vi "ClassPanel.vi"(8 "error in (no error)":errorcluster caption="entrée d'erreur (pas d'erreur)", 11 "ThorKDC101.lvclass":refnum<class "ThorKDC101.lvclass">) -> (0 "error out":errorcluster caption="sortie d'erreur", 3 "ThorKDC101.lvclass Out":refnum<class "ThorKDC101.lvclass">)   [LabVIEW 2019, in "ThorKDC101.lvclass"]
uses:
  ThorKDC101.lvclass
  C:/Programmes Labview/LabScanV1A/DevicesClass/BaseDevice/BaseDevice.lvclass
  BaseDevice/ClassQueueMess.ctl
  ThorKDC101.lvclass/ThorKDC101.ctl
  BaseDevice/Accessor/GetClassEvent.vi
panel:
  in  "Home":bool caption="MiseAJour"
  out "ActPos(Deg)":dbl=60.0 caption="ActPos(deg)" min=0.1 step=0.1 format="%#.1f"
  in  "Con/Disc.":bool
  out "InstrName":string
  out "Homed":bool
  out "Moving":bool
  in  "MainProgQ":refnum<queue>
  in  "MainProgQEvent":refnum<user-event>
  in  "Acq":bool
  in  "Stop":bool
  in  "StopMove":bool caption="MiseAJour"
  in  "Position(Deg)":dbl=60.0 caption="Position(deg)" format="%#.1f"
  out "Init Program":bool
  # "this MUST labeled with class name"
  # "this MUST be present and labeled \"Stop\" and \"Acq\""
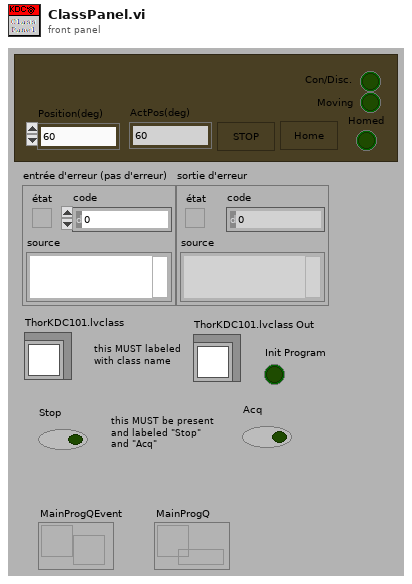
[diagram p1: front panel]
types:
  T1 = typedef "ClassQueueMess.ctl" = u16
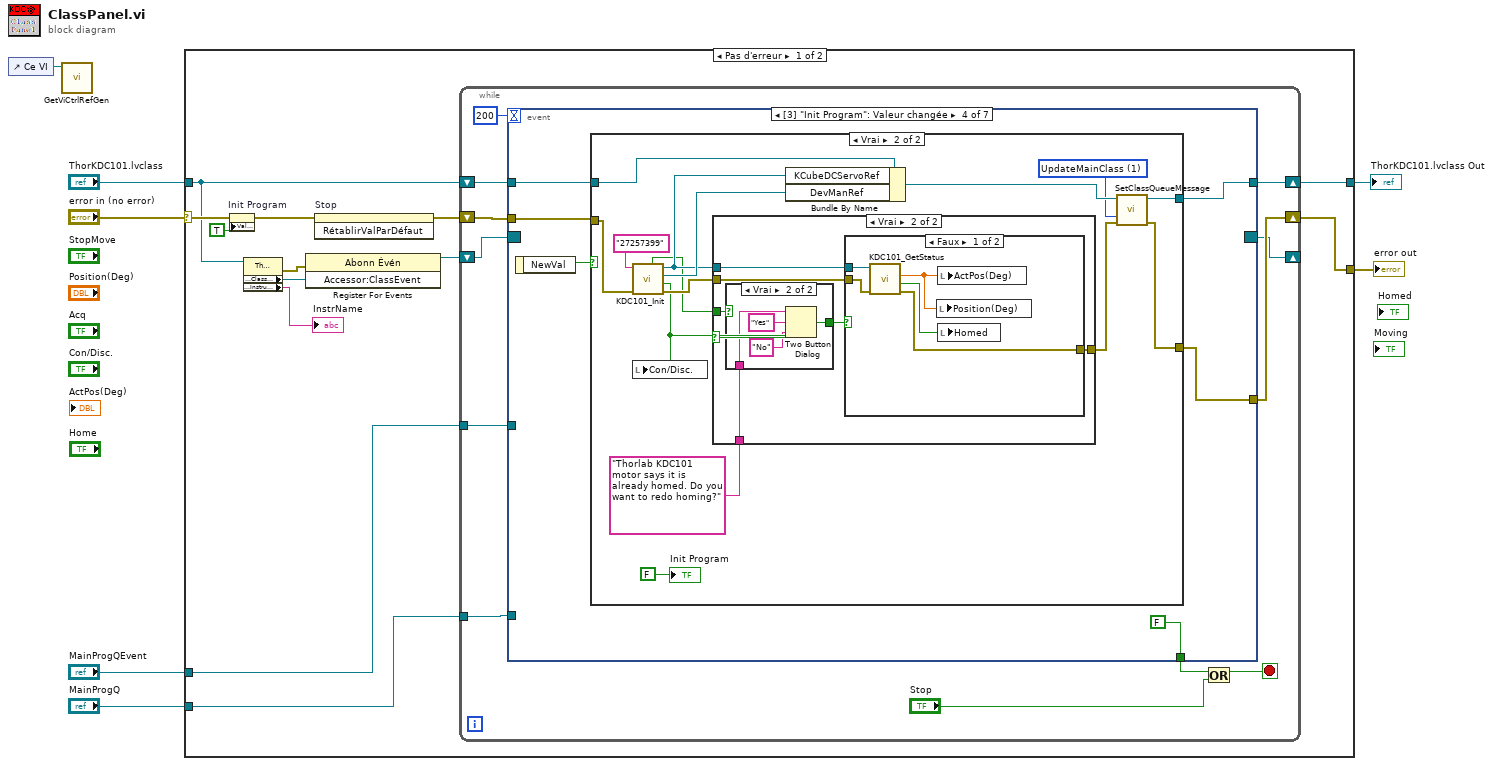
[diagram p0: block diagram]
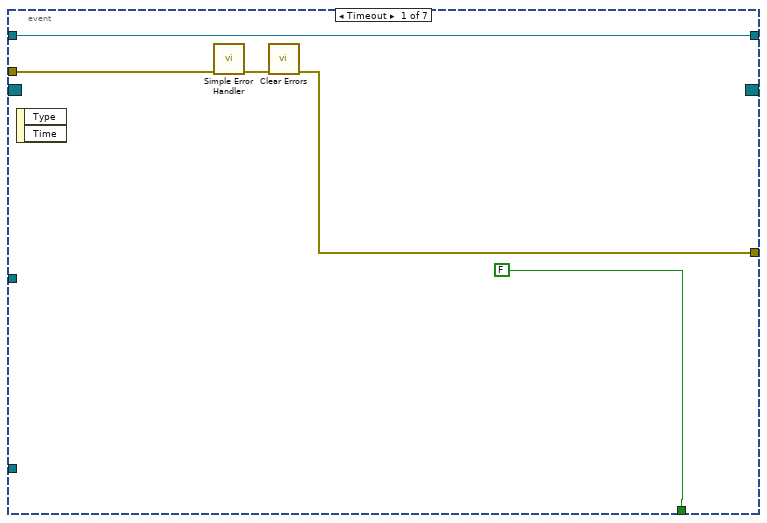
[diagram p2: hidden frame]
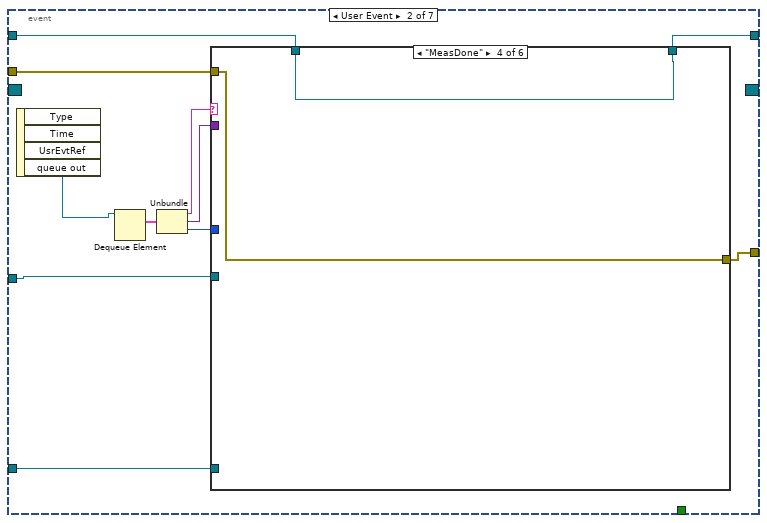
[diagram p3: hidden frame]
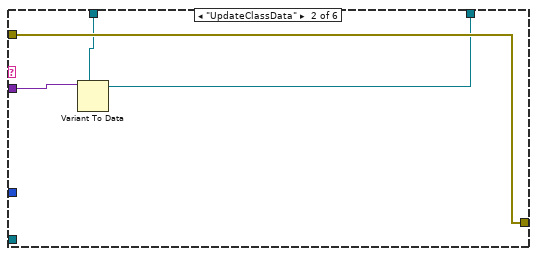
[diagram p5: hidden frame]
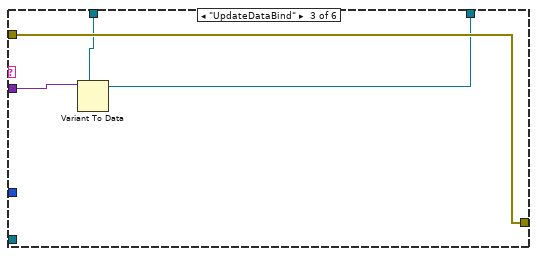
[diagram p6: hidden frame]
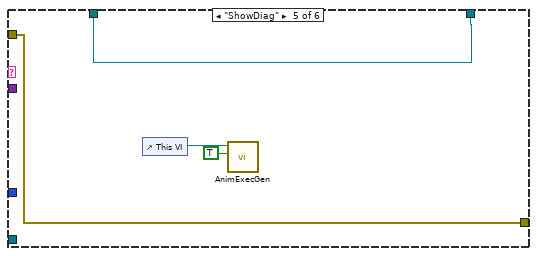
[diagram p7: hidden frame]
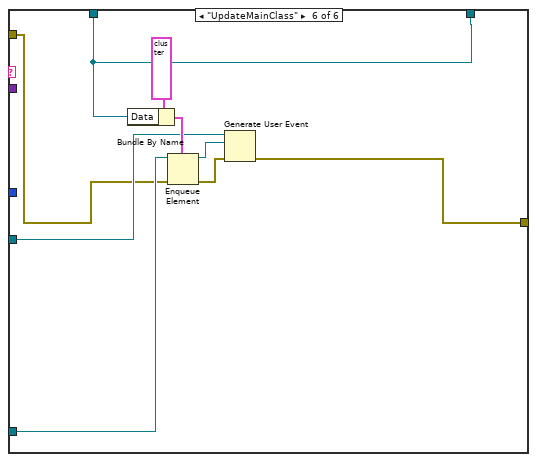
[diagram p8: hidden frame]
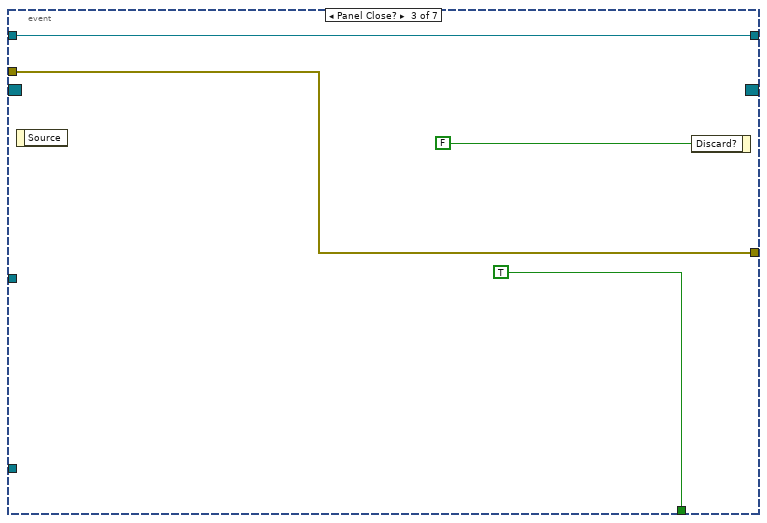
[diagram p9: hidden frame]
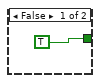
[diagram p12: hidden frame]
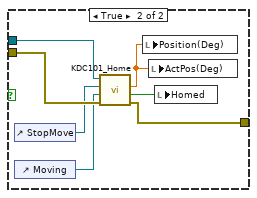
[diagram p13: hidden frame]
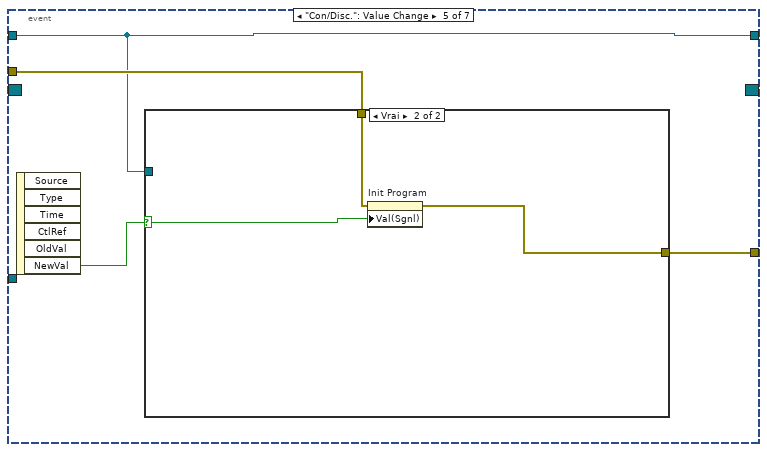
[diagram p14: hidden frame]
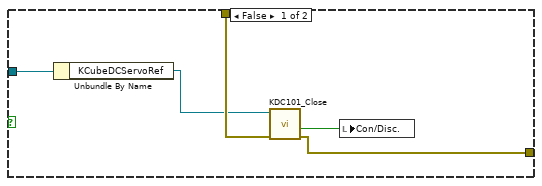
[diagram p15: hidden frame]
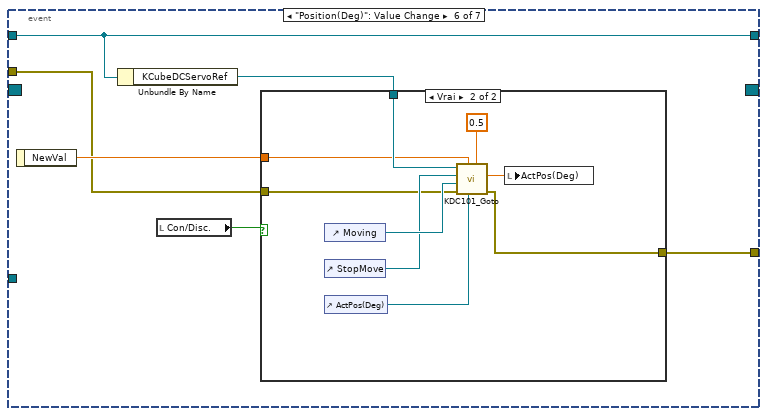
[diagram p16: hidden frame]
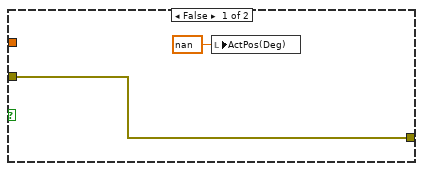
[diagram p17: hidden frame]
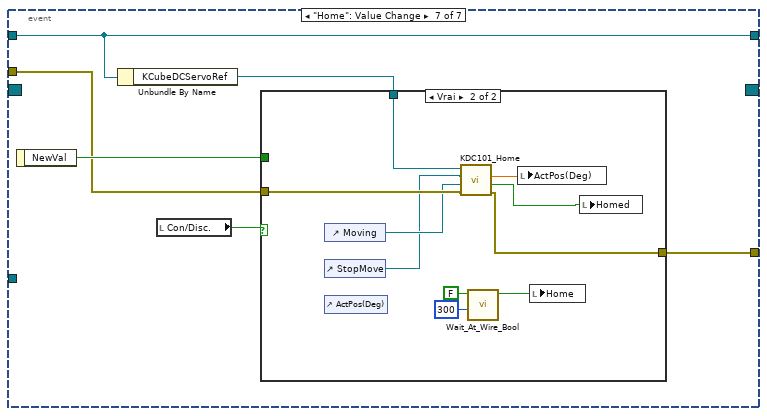
[diagram p18: hidden frame]
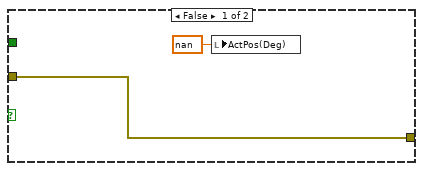
[diagram p19: hidden frame]
diagram:
  n1 = control-ref of="Ce VI"() -> (w1:refnum<vi>)
  n2 = call <userlib>:"GetViCtrlRefGen.vi"("VIRef"=w1) -> ()  [unwired: 8 in, 3 out]
  n3 = case shown="Pas d'erreur" "error in (no error)" {
    selector: "error in (no error)" -> [w17 w173]
    tunnel: [w20 w173] -> w6
    tunnel: "ThorKDC101.lvclass" -> [w12 w172]
    tunnel: [w18 w172] -> w4
    tunnel: "MainProgQEvent" -> [w10 _]
    tunnel: "MainProgQ" -> [w9 _]
    frame No Error {
      n4 = property on="Init Program" class="Bool (strict)"(error in=w17, "Val(Sgnl)"=TRUE ("Valeur (Signalisation)")) -> (error out=w16:errorcluster)  [unwired: 1 in, 1 out]
      n5 = property class="ThorKDC101.lvclass"(reference=w12) -> (error out=w14:errorcluster, "Accessor:ClassEvent"=w13:refnum<user-event>, "Accessor:InstrumentName"=→"InstrName":string)  [unwired: 1 in, 1 out]
      n6 = register-events(error in=w14, w13) -> (reference out=w11:refnum<event-registration>)  [unwired: 1 in, 1 out]
      n7 = invoke on="Stop" class="Bool (strict)" method="RétablirValParDéfaut"(error in=w16) -> (error out=w15:errorcluster)  [unwired: 2 in, 2 out]
      n8 = while {
        shift-right: [w30] -> w20
        shift-left: w15 -> [w31]
        shift-right: [w27] -> w18
        shift-left: w12 -> [w29]
        shift-right: [w23] -> _
        shift-left: w11 -> [w24]
        tunnel: w10 -> [w22]
        tunnel: w9 -> [w21]
        stop <- w26 stop-if-true
        n9 = event shown="[3] \"Init Program\": Valeur changée" {
          selector: w24 -> [_ _ _ _ _ _ _]
          dyn-events: [_ _ _ _ _ _ _] -> w23
          timeout: 200 -> [_ _ _ _ _ _ _]
          tunnel: w31 -> [w35 w47 w75 w82 w127 w139 w156]
          tunnel: [w33 w41 w75 w79 w126 w138 w155] -> w30
          tunnel: w29 -> [w36 w48 w74 w80 w125 w142 w159]
          tunnel: [FALSE _ TRUE FALSE _ _ _] -> w28
          tunnel: [w36 w40 w74 w78 w125 w142 w159] -> w27
          tunnel: w22 -> [_ w39 _ _ _ _ _]
          tunnel: w21 -> [_ w38 _ _ _ _ _]
          event Timeout {
            n10 = event-data() -> ()  [unwired: 1 in, 2 out]
            n11 = call <vilib>:"Simple Error Handler.vi"("error in (no error)"=w35) -> ("error out"=w34:errorcluster)  [unwired: 4 in, 4 out]
            n12 = call <vilib>:"Clear Errors.vi"("error in (no error)"=w34) -> ("error out"=w33:errorcluster)  [unwired: 5 in, 1 out]
          }
          event User Event {
            n13 = event-data() -> ("queue out"=w45:refnum<queue>)  [unwired: 1 in, 3 out]
            n14 = Dequeue Element(queue=w45) -> (element=w46:cluster{"Message":string, "Data":variant, i32})  [unwired: 2 in, 3 out]
            n15 = Unbundle(w46) -> ("Message"=w44:string, "Data"=w43:variant, w42:i32)
            n16 = case shown="\"MeasDone\"" w44 {
              tunnel: w47 -> [w50 w54 w58 w59 w63 w66]
              tunnel: w43 -> [_ w53 w57 _ _ _]
              tunnel: w48 -> [w49 w52 w56 w60 w64 w69]
              tunnel: [w49 w51 w55 w60 w64 w69] -> w40
              tunnel: [w50 w54 w58 w59 w63 w65] -> w41
              tunnel: w42 -> [_ _ _ _ _ _]
              tunnel: w39 -> [_ _ _ _ _ w68]
              tunnel: w38 -> [_ _ _ _ _ w67]
              frame Default {
              }
              frame "UpdateClassData" {
                n17 = Variant To Data(type=w52, Variant=w53) -> (data=w51:refnum<class "ThorKDC101.lvclass">)  [unwired: 1 in, 1 out]
              }
              frame "UpdateDataBind" {
                n18 = Variant To Data(type=w56, Variant=w57) -> (data=w55:refnum<class "ThorKDC101.lvclass">)  [unwired: 1 in, 1 out]
              }
              frame "MeasDone" {
              }
              frame "ShowDiag" {
                n19 = control-ref of="This VI"() -> (w62:refnum<vi>)
                n20 = call <userlib>:"AnimExecGen.vi"("Animer l'exécution ?"=TRUE, "ViRef"=w62) -> ()  [unwired: 9 in, 1 out]
              }
              frame "UpdateMainClass" {
                n21 = Bundle By Name(cluster=cluster{"Message":string, "Data":variant, i32} {"Message"="", "Data"=variant, 0} ("élément"), "Data"=w69) -> (w70:cluster{"Message":string, "Data":variant, i32})
                n22 = Enqueue Element(queue=w67, element=w70, error in (no error)=w66) -> (queue out=w73:refnum<queue>, error out=w72:errorcluster)  [unwired: 1 in, 1 out]
                n23 = Generate User Event(user event=w68, event data cluster=w73, error in=w72) -> (error out=w65:errorcluster)  [unwired: 1 in, 1 out]
              }
            }
          }
          event Panel Close? {
            n24 = event-data() -> ()  [unwired: 1 in, 1 out]
            n25 = event-data("Discard?"=FALSE ("Rejeter ?")) -> ()  [unwired: 1 in, 1 out]
          }
          event "Init Program": Value Change {
            n26 = event-data() -> ("NewVal"=w83:bool)  [unwired: 1 in]
            n27 = case shown="Vrai" w83 {
              tunnel: w82 -> [w85 w95]
              tunnel: [w85 w94] -> w79
              tunnel: w80 -> [w84 w89]
              tunnel: [w84 w93] -> w78
              frame False {
              }
              frame True {
                w96 = T1 1 items=["UpdateClassData", "UpdateMainClass", "UpdateDataBind", "ReInitDevice", "Custom", "ClosePan"] ("Menu déroulant")
                n28 = call <userlib>:"KDC101_Init.vi"("error in (no error)"=w95, "serialNo"="27257399") -> ("error out"=w92:errorcluster, "Connected"=w88:bool, "DevManRef"=w98:refnum<k24>, "KCubeDCServoRef"=w91:refnum<k24>, "IsHomed"=w87:bool)  [unwired: 4 in, 1 out]
                n29 = local write "Con/Disc."(w88) -> ()
                n30 = case shown="Vrai" w88 {
                  tunnel: w92 -> [w101 w107]
                  tunnel: w91 -> [_ w106]
                  tunnel: [w101 w105] -> w90
                  tunnel: w87 -> [_ w102]
                  tunnel: "Thorlab KDC101 motor says it is already homed. Do you want to redo homing?" -> [_ w103]
                  frame False {
                  }
                  frame True {
                    n31 = case shown="Vrai" w102 {
                      tunnel: [TRUE w112] -> w104
                      tunnel: w103 -> [_ w111]
                      frame False {
                      }
                      frame True {
                        n32 = Two Button Dialog(message=w111, 1:"No" ("Nom du bouton F (\"Annuler\")"), 2:"Yes" ("Nom du bouton V (\"OK\")")) -> (T button?=w112:bool)
                      }
                    }
                    n33 = case shown="Faux" w104 {
                      tunnel: w107 -> [w116 w124]
                      tunnel: w106 -> [w117 w121]
                      tunnel: [w115 w119] -> w105
                      frame False {
                        n34 = call <userlib>:"KDC101_GetStatus.vi"("error in (no error)"=w116, "KCubeDCServoRef"=w117) -> ("error out"=w115:errorcluster, "Homed"=w114:bool, "ActPos(Deg)"=w113:dbl)  [unwired: 5 in, 2 out]
                        n35 = local write "Position(Deg)"(w113) -> ()
                        n36 = local write "ActPos(Deg)"(w113) -> ()
                        n37 = local write "Homed"(w114) -> ()
                      }
                      frame True {
                        n38 = control-ref of="StopMove"() -> (w122:refnum<vi>)
                        n39 = control-ref of="Moving"() -> (w123:refnum<vi>)
                        n40 = call <userlib>:"KDC101_Home.vi"("error in (no error)"=w124, "MovingRef"=w123, "StopRef"=w122, "KCubeDCServoRef"=w121) -> ("error out"=w119:errorcluster, "Homed"=w120:bool, "ActPos(Deg)"=w118:dbl)  [unwired: 4 in, 1 out]
                        n41 = local write "Position(Deg)"(w118) -> ()
                        n42 = local write "ActPos(Deg)"(w118) -> ()
                        n43 = local write "Homed"(w120) -> ()
                      }
                    }
                  }
                }
                n44 = Bundle By Name(cluster=w89, "KCubeDCServoRef"=w91, "DevManRef"=w98) -> (w97:refnum<class "ThorKDC101.lvclass">)
                n45 = call-dynamic "SetClassQueueMessage.vi"("ErrorIn(No Error)"=w90, "Menu déroulant"=w96, "DefaultDev.lvclass"=w97) -> ("sortie d'erreur"=w94:errorcluster, "DefaultDev.lvclass Out"=w93:refnum<class "ThorKDC101.lvclass">)  [unwired: 7 in]
                "Init Program" <- FALSE
              }
            }
          }
          event "Con/Disc.": Value Change {
            n46 = event-data() -> ("NewVal"=w128:bool)  [unwired: 1 in, 5 out]
            n47 = case shown="Vrai" w128 {
              selector: w128 -> [_ w136]
              tunnel: w127 -> [w133 w135]
              tunnel: [w130 w134] -> w126
              tunnel: w125 -> [w132 _]
              frame False {
                n48 = Unbundle By Name(w132) -> ("KCubeDCServoRef"=w131:refnum<k24>)
                n49 = call <userlib>:"KDC101_Close.vi"("error in (no error)"=w133, "KCubeDCServoRefIn"=w131) -> ("error out"=w130:errorcluster, "Connected"=w129:bool)  [unwired: 7 in, 1 out]
                n50 = local write "Con/Disc."(w129) -> ()
              }
              frame True {
                n51 = property on="Init Program" class="Bool (strict)"(error in=w135, "Val(Sgnl)"=w136) -> (error out=w134:errorcluster)  [unwired: 1 in, 1 out]
              }
            }
          }
          event "Position(Deg)": Value Change {
            n52 = event-data() -> ("NewVal"=w140:dbl)  [unwired: 1 in]
            n53 = Unbundle By Name(w142) -> ("KCubeDCServoRef"=w141:refnum<k24>)
            n54 = local read "Con/Disc."() -> (w137:bool)
            n55 = case shown="Vrai" w137 {
              tunnel: w141 -> [_ w153]
              tunnel: w140 -> [_ w151]
              tunnel: w139 -> [w144 w147]
              tunnel: [w144 w146] -> w138
              frame False {
                n56 = local write "ActPos(Deg)"(nan ("ActPos(Deg)")) -> ()
              }
              frame True {
                n57 = control-ref of="Moving"() -> (w150:refnum<vi>)
                n58 = control-ref of="StopMove"() -> (w149:refnum<vi>)
                n59 = control-ref of="ActPos(Deg)"() -> (w148:refnum<vi>)
                n60 = call <userlib>:"KDC101_Goto.vi"("ErrRange(deg)"=0.5, "PositionRef"=w148, "Position(deg)"=w151, "error in (no error)"=w147, "MovingRef"=w150, "StopRef"=w149, "KCubeDCServoRef"=w153) -> ("error out"=w146:errorcluster, "PositionOut(deg)"=w145:dbl)  [unwired: 1 in, 2 out]
                n61 = local write "ActPos(Deg)"(w145) -> ()
              }
            }
          }
          event "Home": Value Change {
            n62 = event-data() -> ("NewVal"=w157:bool)  [unwired: 1 in]
            n63 = Unbundle By Name(w159) -> ("KCubeDCServoRef"=w158:refnum<k24>)
            n64 = local read "Con/Disc."() -> (w154:bool)
            n65 = case shown="Vrai" w154 {
              tunnel: w158 -> [_ w167]
              tunnel: w157 -> [_ _]
              tunnel: w156 -> [w161 w170]
              tunnel: [w161 w171] -> w155
              frame False {
                n66 = local write "ActPos(Deg)"(nan ("ActPos(Deg)")) -> ()
              }
              frame True {
                n67 = control-ref of="Moving"() -> (w169:refnum<vi>)
                n68 = control-ref of="StopMove"() -> (w168:refnum<vi>)
                n69 = control-ref of="ActPos(Deg)"() -> ()  [unwired: 1 out]
                n70 = call <userlib>:"KDC101_Home.vi"("error in (no error)"=w170, "MovingRef"=w169, "StopRef"=w168, "KCubeDCServoRef"=w167) -> ("error out"=w171:errorcluster, "Homed"=w165:bool, "ActPos(Deg)"=w166:dbl)  [unwired: 4 in, 1 out]
                n71 = call <userlib>:"Wait_At_Wire_Bool.vi"("Wait (ms)"=u32 300, "error in (no error)"=FALSE) -> ("error out"=w162:bool)  [unwired: 7 in, 2 out]
                n72 = local write "ActPos(Deg)"(w166) -> ()
                n73 = local write "Home"(w162) -> ()
                n74 = local write "Homed"(w165) -> ()
              }
            }
          }
        }
        n75 = Or(x=w28, y="Stop") -> (x .or. y?=w26:bool)
      }
    }
    frame Error {
    }
  }
  "error out" <- w6
  "ThorKDC101.lvclass Out" <- w4
